vi "GCLILauncher.vi"   [LabVIEW 2019, in "MicronTemplateService.lvlib"]
doc: "Launcher VI to get arguments from G-CLI and start the service in LabVIEW source code.\n\nTo manually launch, directly use Main.vi"
uses:
  MicronTemplateService.lvlib
  <vilib>/Wiresmith Technology/G CLI/CLI Class/CLI.lvclass
panel:
  # "Launcher VI to get arguments from G-CLI  and start the service in LabVIEW source code.\n\nTo manually launch, directly use Main.vi"
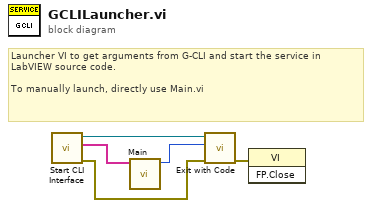
[diagram p0: block diagram]
diagram:
  # "Launcher VI to get arguments from G-CLI and start the service in LabVIEW source code.\n\nTo manually launch, directly use Main.vi"
  n1 = call <vilib>:"Start CLI Interface.vi"() -> ("error out"=w2:errorcluster, "Custom Parameters"=w5:string[], "CLI out"=w3:refnum<class "CLI.lvclass">)  [unwired: 8 in, 1 out]
  n2 = call "Main.vi"("Args"=w5) -> ("Return Status"=w4:i32)  [unwired: 9 in, 1 out]
  n3 = call <vilib>:"Exit with Code.vi"("error in (no error)"=w2, "Exit Code (0)"=w4, "CLI in"=w3) -> ("error out"=w1:errorcluster)  [unwired: 8 in]
  n4 = invoke class="VI" method="FP.Close"(error in=w1) -> ()  [unwired: 2 in, 3 out]
